vi "stop.vi"(8 "error in (no error)":errorcluster, 11 "FPGAWrapperRK120511Fiber_Spiral in":refnum<class "FPGAWrapperRK110512Fiber_Spiral.lvclass">) -> (0 "error out":errorcluster, 3 "FPGAWrapperRK120511Fiber_Spiral out":refnum<class "FPGAWrapperRK110512Fiber_Spiral.lvclass">)   [LabVIEW 2010, in "FPGAWrapperRK110512Fiber_Spiral.lvclass"]
uses:
  FPGAWrapperRK110512Fiber_Spiral.lvclass
  <vilib>/rvi/interface/nirviReadWriteControl/nirviReadWriteControl.xnode
  FPGA_VI_Reference.ctl
  <vilib>/rvi/interface/common/niFpgaNodeNameForErrorReporting.ctl
  <vilib>/rvi/errors/niLvFpgaWhatHappensToTopLevelVI.ctl
  <vilib>/Utility/error.llb/Error Cluster From Error Code.vi
  <vilib>/rvi/errors/niLvFpgaAdjustHostInterfaceError.vi
  NiFpgaLv.dll
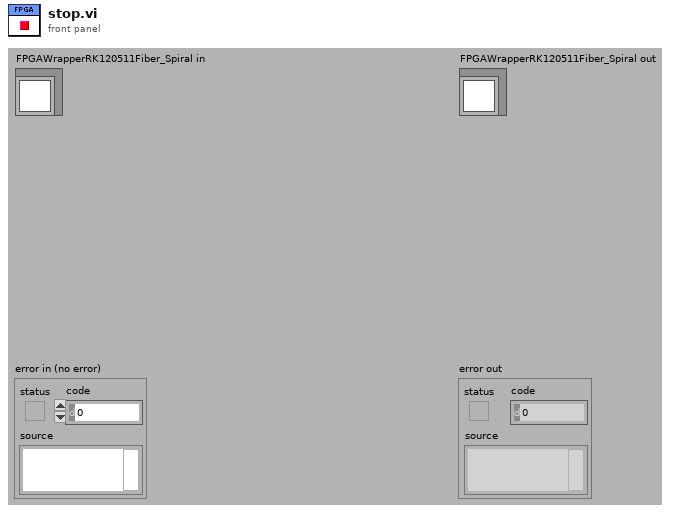
[diagram p1: front panel]
types:
  T1 = typedef "niFpgaNodeNameForErrorReporting.ctl" = enum16{"Open FPGA VI Reference", "Read/Write Control", "Invoke Method: Abort", "Invoke Method: Acknowledge IRQ", "Invoke Method: Download", "Invoke Method: FIFO.Configure", "Invoke Method: FIFO.Read", "Invoke Method: FIFO.Start", "Invoke Method: FIFO.Stop", "Invoke Method: FIFO.Write", "Invoke Method: Reset", "Invoke Method: Run", "Invoke Method: Wait on IRQ", "Close FPGA VI Reference"}
  T2 = typedef "niLvFpgaWhatHappensToTopLevelVI.ctl" = enum16{"top level VI scripted behind XNode", "top level VI inlined behind XNode"}
  T3 = typedef "FPGAWrapperRK110512Fiber_Spiral.lvclass/FPGA_VI_Reference.ctl" = refnum<k20>
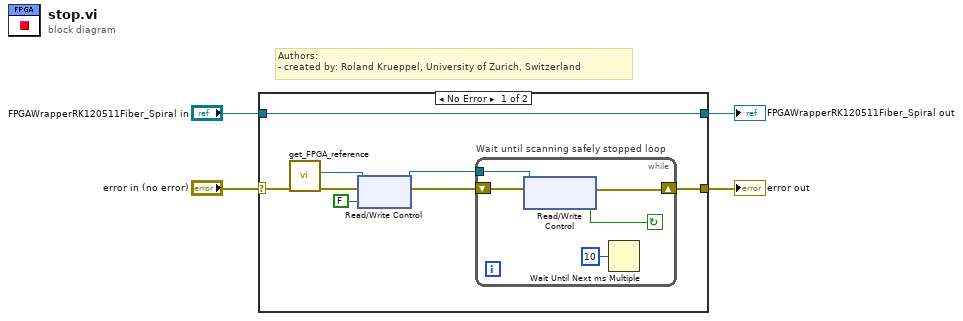
[diagram p0: block diagram]
diagram:
  # "Authors: \n- created by: Roland Krueppel, University of Zurich, Switzerland"
  n1 = case shown="No Error" "error in (no error)" {
    selector: "error in (no error)" -> [w12 w100]
    tunnel: "FPGAWrapperRK120511Fiber_Spiral in" -> [w8 w101]
    tunnel: [w8 w101] -> w2
    tunnel: [w6 w100] -> w1
    frame No Error {
      n2 = call "get_FPGA_reference.vi"("error in (no error)"=w12) -> ("error out"=w11:errorcluster, "FPGA VI Reference"=w10:T3)  [unwired: 8 in, 1 out]
      n3 = xnode "Read/Write Control"("FPGA VI Reference In"=w10, "error in"=w11, "Scan"=FALSE) -> ("FPGA VI Reference Out"=w5:T3, "error out"=w7:errorcluster)
      n4 = while "Wait until scanning safely stopped loop" {
        shift-right: [w14] -> w6
        shift-left: w7 -> [w16]
        tunnel: w5 -> [w17]
        stop <- w15 continue-if-true
        n5 = xnode "Read/Write Control"("FPGA VI Reference In"=w17, "error in"=w16) -> ("error out"=w14:errorcluster, "Scanning?"=w15:bool)  [unwired: 1 out]
        n6 = Wait Until Next ms Multiple(millisecond multiple=u32 10) -> ()  [unwired: 1 out]
      }
    }
    frame Error {
    }
  }
  "error out" <- w1
  "FPGAWrapperRK120511Fiber_Spiral out" <- w2
